vi "To String (Null).vi"(11 "error in (no error)":errorcluster) -> (4 "String":string, 15 "error out":errorcluster)   [LabVIEW 2020, in "Variant JSON API.lvlib"]
doc: "Flattens the given JSON data to a string."
uses:
  Variant JSON API.lvlib
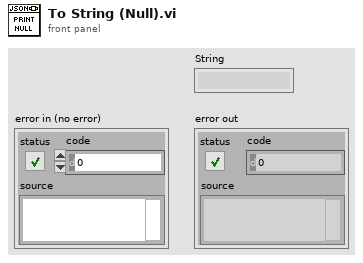
[diagram p1: front panel]
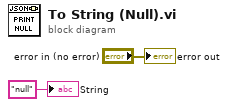
[diagram p0: block diagram]
diagram:
  "String" <- "null" ("String")
  "error out" <- "error in (no error)"
